vi "Fission Reactor.vi"(5 "Coolant Type":enum16{"Water", "Sodium"}(ring), 6 "Burn Rate (mB/t)":dbl, 7 "Activate":bool, 8 "Efficiency (η)":dbl=4.0 min=4.0 max=18.0 step=1.0, 9 "Height (m)":i32=4 min=4 max=18 step=1, 10 "Width (m)":i32=3 min=3 max=18 step=1, 11 "Length (m)":i32=3 min=3 max=18 step=1) -> (0 "Real Heating Rate (mB/t)":u32, 1 "Heating Rate (mB/t)":u32, 2 "Actual Burn Rate (mB/t)":dbl(knob) scale=0.0..1.0, 3 "Computed Build Properties":T1)   [LabVIEW 2023]
uses:
  Reactor Build Properties.ctl
panel:
  out "Heating Rate (mB/t)":dbl(slide) scale=0.0..20000.0 scale format="%#_6p"
  # "Fission Reactor Properties"
  # "Fission Reactor Control"
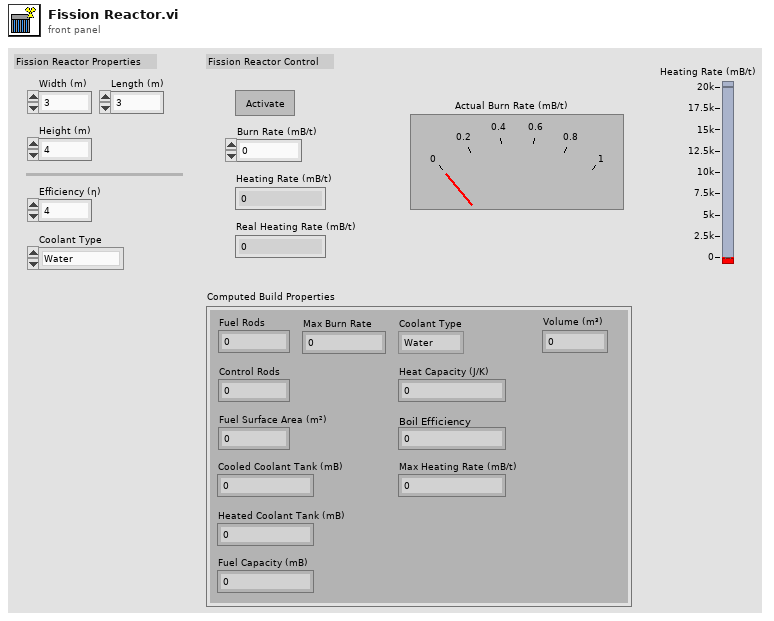
[diagram p1: front panel]
types:
  T1 = typedef "Reactor Build Properties.ctl" = cluster{"Fuel Rods":i32, "Control Rods":i32, "Volume (m³)":i32, "Fuel Surface Area (m²)":i32, "Cooled Coolant Tank (mB)":i32, "Fuel Capacity (mB)":i64, "Heat Capacity (J/K)":dbl, "Max Burn Rate":i64, "Max Heating Rate (mB/t)":i64, "Boil Efficiency":dbl, "Coolant Type":enum16{"Water", "Sodium"}, "Heated Coolant Tank (mB)":i64}
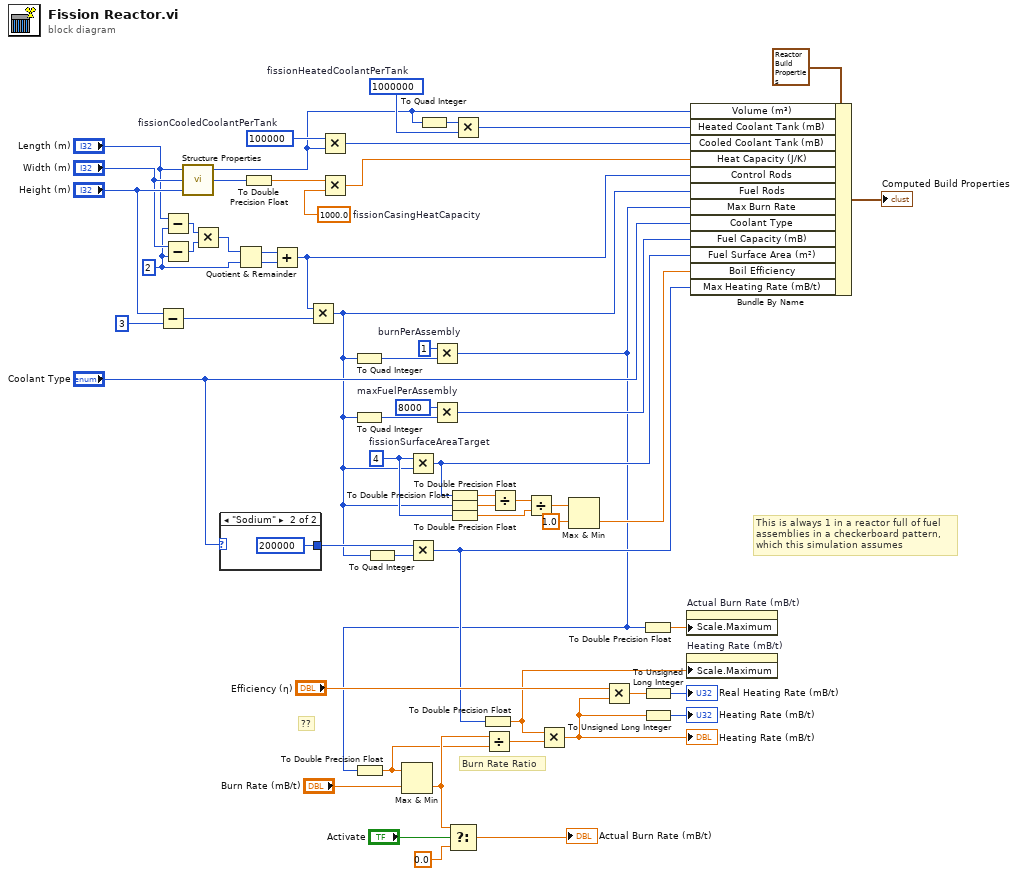
[diagram p0: block diagram]
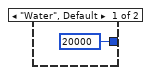
[diagram p2: hidden frame]
diagram:
  w3 = i64 1  # burnPerAssembly
  w13 = i64 1000000  # fissionHeatedCoolantPerTank
  w45 = 1000.0  # fissionCasingHeatCapacity
  w8 = 4  # fissionSurfaceAreaTarget
  w49 = i64 8000  # maxFuelPerAssembly
  w47 = 100000  # fissionCooledCoolantPerTank
  w33 = 2 ("y")
  # "??"
  # "This is always 1 in a reactor full of fuel\nassemblies in a checkerboard pattern,\nwhich this simulation assumes"
  # "Burn Rate Ratio"
  n1 = Subtract(x="Height (m)", y=3) -> (x-y=w57:i32)
  n2 = Subtract(x="Length (m)", y=w33) -> (x-y=w32:i32)
  n3 = Subtract(x="Width (m)", y=w33) -> (x-y=w31:i32)
  n4 = call "Structure Properties.vi"("Length"="Length (m)", "Width"="Width (m)", "Height"="Height (m)") -> ("Volume"=w12:i32, "Casing"=w46:i32)  [unwired: 2 in, 3 out]
  n5 = Multiply(x=w32, y=w31) -> (x*y=w30:i32)
  n6 = case shown="\"Sodium\"" "Coolant Type" {
    tunnel: [i64 20000 ("x") i64 200000 ("x")] -> w17
    frame "Water", Default {
    }
    frame "Sodium" {
    }
  }
  n7 = Quotient & Remainder(x=w30, y=w33) -> (x-y*floor(x/y)=w56:i32, floor(x/y)=w55:i32)
  n8 = To Double Precision Float(number=w46) -> (double precision float=w16:dbl)
  n9 = Add(x=w56, y=w55) -> (x+y=w27:i32)
  n10 = Multiply(x=w27, y=w57) -> (x*y=w2:i32)
  n11 = Multiply(x=w47, y=w12) -> (x*y=w29:i32)
  n12 = Multiply(x=w16, y=w45) -> (x*y=w28:dbl)
  n13 = To Quad Integer(1:w2) -> (0:w4:i64)
  n14 = To Quad Integer(1:w2) -> (0:w9:i64)
  n15 = To Quad Integer(1:w2) -> (0:w6:i64)
  n16 = Multiply(x=w8, y=w2) -> (x*y=w24:i32)
  n17 = Multiply(x=w17, y=w6) -> (x*y=w15:i64)
  n18 = To Quad Integer(1:w12) -> (0:w11:i64)
  n19 = Multiply(x=w3, y=w4) -> (x*y=w1:i64)
  n20 = To Double Precision Float(number=w1) -> (double precision float=w42:dbl)
  n21 = Max & Min(x=w42, y="Burn Rate (mB/t)") -> (min(x,y)=w43:dbl)  [unwired: 1 out]
  n22 = Multiply(x=w49, y=w9) -> (x*y=w10:i64)
  n23 = Select(t=w43, s="Activate", f=0.0) -> (s? t:f=→"Actual Burn Rate (mB/t)":dbl)
  n24 = To Double Precision Float(number=w24) -> (double precision float=w23:dbl)
  n25 = To Double Precision Float(number=w2) -> (double precision float=w22:dbl)
  n26 = To Double Precision Float(number=w8) -> (double precision float=w7:dbl)
  n27 = Multiply(x=w11, y=w13) -> (x*y=w14:i64)
  n28 = To Double Precision Float(number=w15) -> (double precision float=w36:dbl)
  n29 = Divide(x=w43, y=w42) -> (x/y=w41:dbl)
  n30 = Divide(x=w23, y=w22) -> (x/y=w21:dbl)
  n31 = Divide(x=w21, y=w7) -> (x/y=w19:dbl)
  n32 = Multiply(x=w36, y=w41) -> (x*y=w38:dbl)
  "Heating Rate (mB/t)" <- w38
  n33 = Max & Min(x=w19, y=1.0) -> (min(x,y)=w20:dbl)  [unwired: 1 out]
  n34 = Multiply(x="Efficiency (η)", y=w38) -> (x*y=w40:dbl)
  n35 = To Double Precision Float(number=w1) -> (double precision float=w54:dbl)
  n36 = To Unsigned Long Integer(number=w40) -> (unsigned 32bit integer=→"Real Heating Rate (mB/t)":u32)
  n37 = To Unsigned Long Integer(number=w38) -> (unsigned 32bit integer=→"Heating Rate (mB/t)":u32)
  n38 = property on="Actual Burn Rate (mB/t)" class="Knob (strict)"("Scale.Maximum"=w54) -> ()  [unwired: 2 in, 2 out]
  n39 = property on="Heating Rate (mB/t)" class="Slide (strict)"("Scale.Maximum"=w36) -> ()  [unwired: 2 in, 2 out]
  n40 = Bundle By Name(cluster=T1 {"Fuel Rods"=0, "Control Rods"=0, "Volume (m³)"=0, "Fuel Surface Area (m²)"=0, "Cooled Coolant Tank (mB)"=0, "Fuel Capacity (mB)"=0, "Heat Capacity (J/K)"=0.0, "Max Burn Rate"=0, "Max Heating Rate (mB/t)"=0, "Boil Efficiency"=0.0, "Coolant Type"=enum."Water", "Heated Coolant Tank (mB)"=0} ("Reactor Build Properties"), "Volume (m³)"=w12, "Heated Coolant Tank (mB)"=w14, "Cooled Coolant Tank (mB)"=w29, "Heat Capacity (J/K)"=w28, "Control Rods"=w27, "Fuel Rods"=w2, "Max Burn Rate"=w1, "Coolant Type"="Coolant Type", "Fuel Capacity (mB)"=w10, "Fuel Surface Area (m²)"=w24, "Boil Efficiency"=w20, "Max Heating Rate (mB/t)"=w15) -> (→"Computed Build Properties":T1)
